vi "InitLinkButtons.vi"(5 "rightColumnAlignment":refnum<vi>, 6 "Col1Sec3_Top":refnum<vi>, 7 "leftColumnAlignment":refnum<vi>, 8 "icon array":refnum<vi>[](array[refnum]), 9 "button array":refnum<vi>[][](array[refnum]), 10 "item info array":T1(array[cluster]), 11 "Pnl Refnum":refnum<vi>) -> (3 "Handler info":variant)   [LabVIEW 2009, in "NavScreen.lvlib"]
uses:
  NavScreen.lvlib
  Classes/ClickableText/ClickableText.lvclass
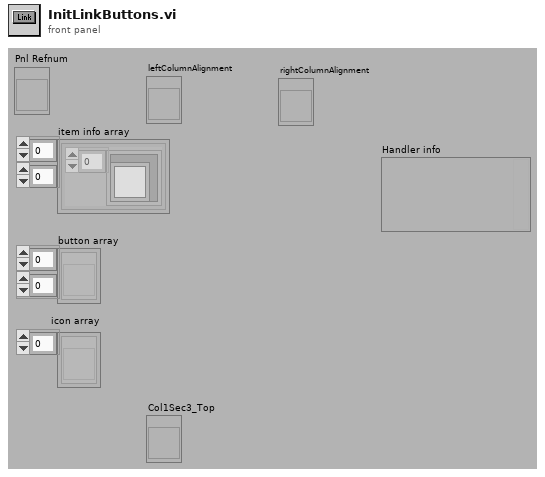
[diagram p1: front panel]
types:
  T1 = cluster{refnum<class "ClickableText.lvclass">[]}[][]
  T2 = typedef "NavScreen.lvlib/ItemData_Type.ctl" = enum16{"None", "Folder", "New Project", "New VI", "Find", "VI", "Project", "New from template", "RT Project Wizard", "PDA Project Wizard", "Control", "Library", "Class", "XControl", "Runtime menu"}
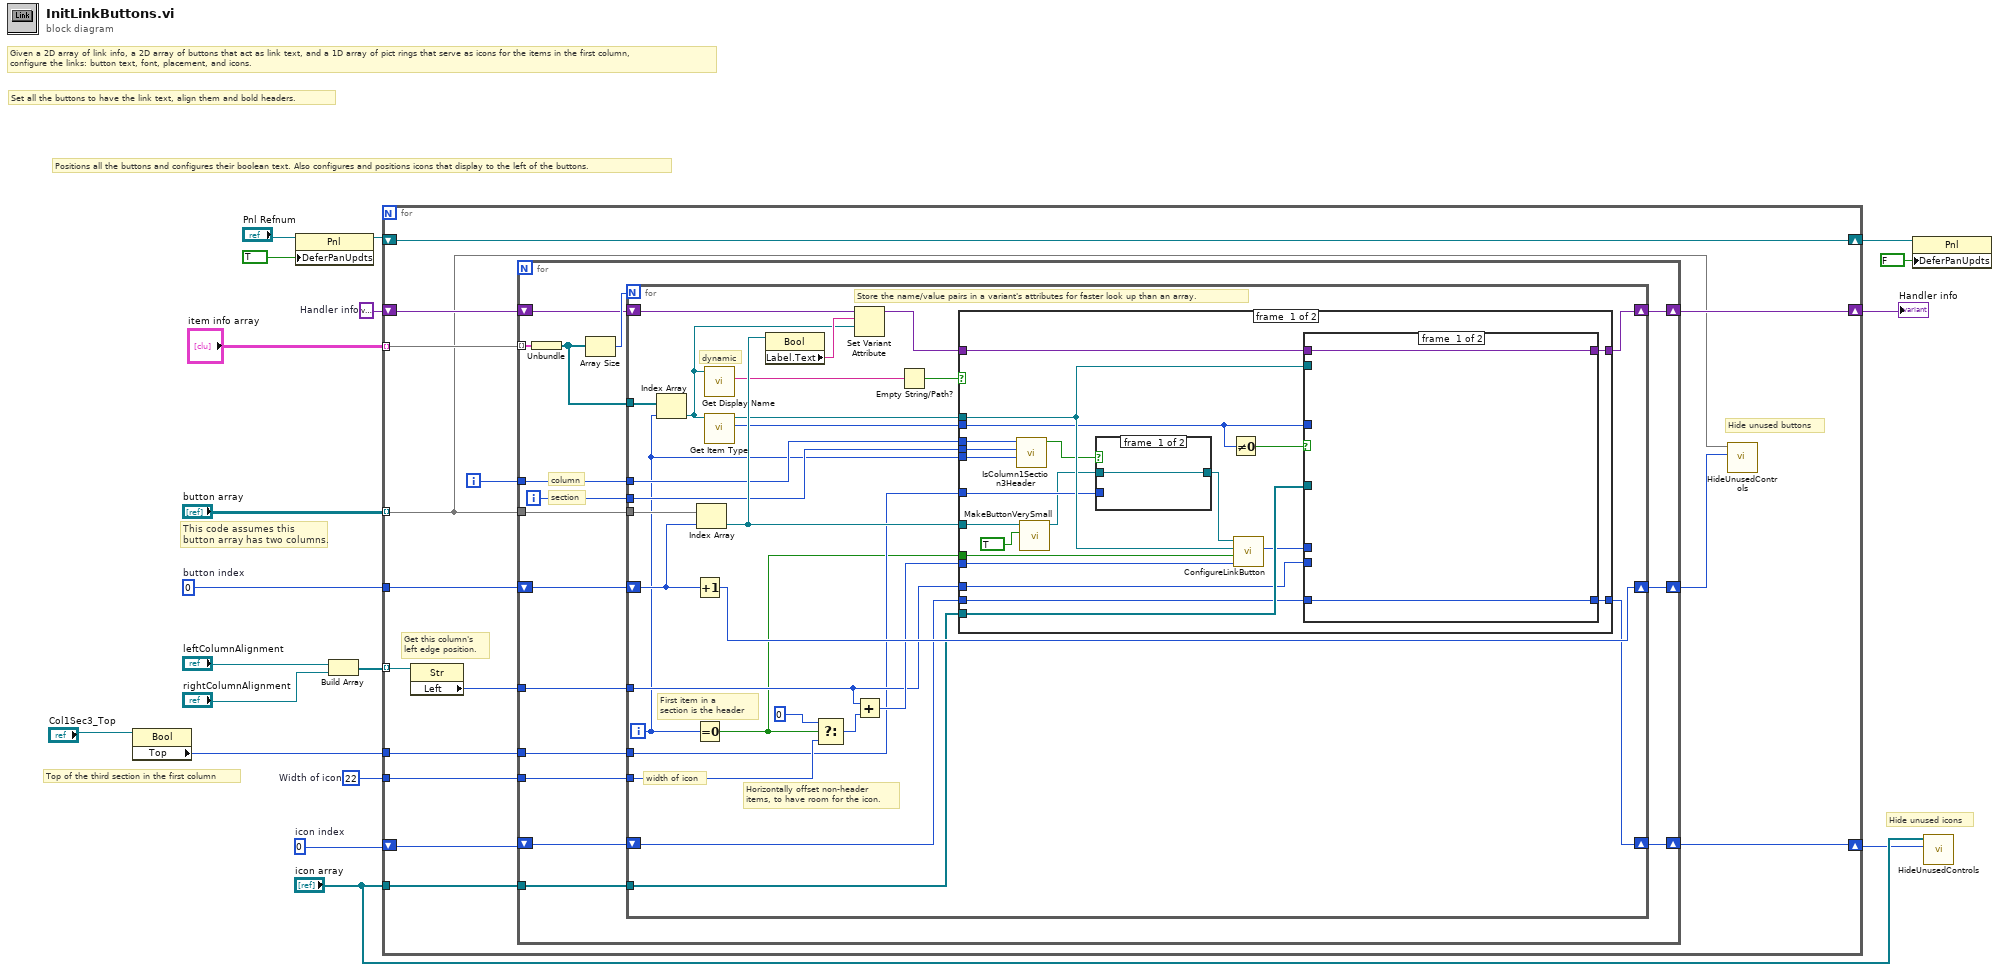
[diagram p0: block diagram]
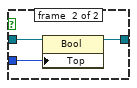
[diagram p2: hidden frame]
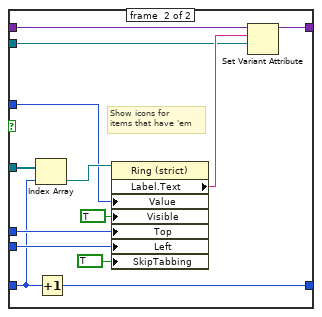
[diagram p3: hidden frame]
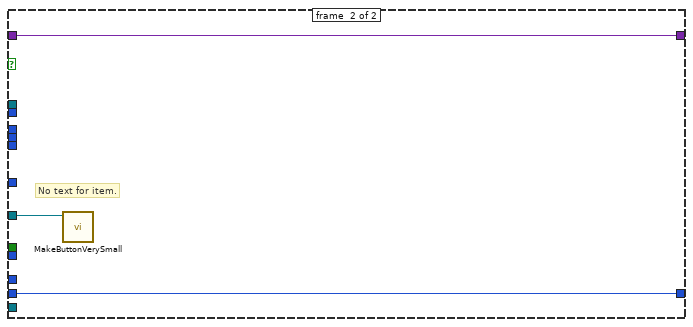
[diagram p4: hidden frame]
diagram:
  w2 = 0  # button index
  w4 = variant  # Handler info
  w9 = 22  # Width of icon
  w13 = 0  # icon index
  # "Positions all the buttons and configures their boolean text. Also configures and positions icons that display to the left of the buttons."
  # "Set all the buttons to have the link text, align them and bold headers."
  # "Top of the third section in the first column"
  # "Given a 2D array of link info, a 2D array of buttons that act as link text, and a 1D array of pict rings that serve as icons for the items in the first column,\nconfigure the links: button text, font, placement, and icons."
  # "This code assumes this\nbutton array has two columns."
  # "Hide unused icons"
  n1 = property on="Property Node" class="Bool"(reference="Col1Sec3_Top") -> ("Top"=w7:i32)  [unwired: 1 in, 2 out]
  n2 = property on="Property Node" class="Pnl"(reference="Pnl Refnum", "DeferPanUpdts"=TRUE ("Defer Panel Updates")) -> (reference out=w16:refnum<vi>)  [unwired: 1 in, 1 out]
  n3 = Build Array("leftColumnAlignment", "rightColumnAlignment") -> (w10:refnum<vi>[])
  n4 = for {
    tunnel: "button array" -> [w22] mode=indexing
    tunnel: "item info array" -> [w33] mode=indexing
    tunnel: "icon array" -> [w32]
    shift-right: [w30] -> w3
    shift-left: w4 -> [w31]
    shift-right: [w29] -> w14
    shift-left: w16 -> [w29]
    tunnel: w9 -> [w28]
    shift-right: [w26] -> w5
    shift-left: w13 -> [w27]
    tunnel: w10 -> [w25] mode=indexing
    tunnel: w7 -> [w24]
    tunnel: w2 -> [w20]
    i -> [w23]
    # "Get this column's\nleft edge position."
    # "Hide unused buttons"
    n5 = property on="Property Node" class="Str"(reference=w25) -> ("Left"=w34:i32)  [unwired: 1 in, 2 out]
    n6 = for {
      tunnel: w22 -> [w50]
      tunnel: w33 -> [w39] mode=indexing
      shift-right: [w48] -> w21
      shift-left: w20 -> [w49]
      tunnel: w34 -> [w47]
      shift-right: [w35] -> w30
      shift-left: w31 -> [w36]
      shift-right: [w45] -> w26
      shift-left: w27 -> [w46]
      tunnel: w32 -> [w44]
      tunnel: w28 -> [w43]
      tunnel: w24 -> [w42]
      tunnel: w23 -> [w41]
      i -> [w40]
      # "section"
      # "column"
      n7 = Unbundle(w39) -> (w37:refnum<class "ClickableText.lvclass">[])
      n8 = Array Size(array=w37) -> (size(s)=w38:i32)
      n9 = for {
        N: w38 -> [_]
        tunnel: w37 -> [w71]
        tunnel: w50 -> [w77]
        shift-right: [w75] -> w48
        shift-left: w49 -> [w76]
        tunnel: w47 -> [w66]
        shift-right: [w68] -> w45
        shift-left: w46 -> [w69]
        tunnel: w44 -> [w56]
        tunnel: w43 -> [w67]
        tunnel: w42 -> [w65]
        tunnel: w41 -> [w64]
        tunnel: w40 -> [w63]
        shift-right: [w51] -> w35
        shift-left: w36 -> [w57]
        i -> [w62]
        # "dynamic"
        # "First item in a\nsection is the header"
        # "Store the name/value pairs in a variant's attributes for faster look up than an array."
        # "width of icon"
        # "Horizontally offset non-header\nitems, to have room for the icon."
        n10 = Index Array(array=w71, index=w62) -> (element=w58:refnum<class "ClickableText.lvclass">)
        n11 = Increment(x=w76) -> (x+1=w75:i32)
        n12 = Equal To 0?(x=w62) -> (x = 0?=w54:bool)
        n13 = Index Array(array=w77, index=w76) -> (element=w70:refnum<vi>)
        n14 = call-dynamic "Get Display Name.vi"("ClickableText in"=w58) -> ("localized name"=w61:string)  [unwired: 8 in, 2 out]
        n15 = call "Get Item Type.vi"("ClickableText in"=w58) -> ("DNL_Type"=w60:T2, "ClickableText out"=w53:refnum<class "ClickableText.lvclass">)  [unwired: 8 in, 1 out]
        n16 = property on="Property Node" class="Bool"(reference=w70) -> ("Label.Text"=w59:string)  [unwired: 1 in, 2 out]
        n17 = Select(t=0, s=w54, f=w67) -> (s? t:f=w55:i32)
        n18 = Set Variant Attribute(Variant=w57, name=w59, value=w58) -> (Variant out=w52:variant)  [unwired: 1 in, 2 out]
        n19 = Add(x=w66, y=w55) -> (x+y=w74:i32)
        n20 = Empty String/Path?(string/path=w61) -> (empty?=w72:bool)
        n21 = case shown="False" w72 {
          tunnel: w74 -> [w80 _]
          tunnel: w70 -> [w90 w119]
          tunnel: w54 -> [w83 _]
          tunnel: w56 -> [w97 _]
          tunnel: w60 -> [w96 _]
          tunnel: w69 -> [w94 w120]
          tunnel: [w93 w120] -> w68
          tunnel: w66 -> [w81 _]
          tunnel: w65 -> [w92 _]
          tunnel: w64 -> [w87 _]
          tunnel: w63 -> [w86 _]
          tunnel: w62 -> [w85 _]
          tunnel: w53 -> [w98 _]
          tunnel: w52 -> [w79 w118]
          tunnel: [w78 w118] -> w51
          frame #0 {
            n22 = call "IsColumn1Section3Header.vi"("index 3"=w85, "index 2"=w86, "index 1"=w87) -> ("is col 1 section 3 header?"=w88:bool)  [unwired: 7 in, 1 out]
            n23 = call "MakeButtonVerySmall.vi"("visible"=TRUE ("Visible"), "Link Button 1"=w90) -> ("Link Button 2"=w89:refnum<vi>)  [unwired: 8 in, 1 out]
            n24 = case shown="True" w88 {
              tunnel: w89 -> [w99 w102]
              tunnel: [w99 w101] -> w84
              tunnel: w92 -> [_ w100]
              frame #0 {
              }
              frame #1 {
                n25 = property on="Property Node" class="Bool"(reference=w102, "Top"=w100) -> (reference out=w101:refnum<vi>)  [unwired: 1 in, 1 out]
              }
            }
            n26 = Not Equal To 0?(x=w96) -> (x != 0?=w95:bool)
            n27 = call "ConfigureLinkButton.vi"("Position:Left"=w80, "is section header?"=w83, "GettingStartedWindow.lvlib:ClickableText.lvclass"=w98, "Link Button 1"=w84) -> ("Top"=w82:i32)  [unwired: 6 in, 1 out]
            n28 = case shown="True" w95 {
              tunnel: w96 -> [_ w109]
              tunnel: w97 -> [_ w112]
              tunnel: w94 -> [w104 w110]
              tunnel: [w104 w116] -> w93
              tunnel: w82 -> [_ w115]
              tunnel: w81 -> [_ w114]
              tunnel: w79 -> [w103 w108]
              tunnel: w98 -> [_ w106]
              tunnel: [w103 w105] -> w78
              frame #0 {
              }
              frame #1 {
                # "Show icons for\nitems that have 'em"
                n29 = Index Array(array=w112, index=w110) -> (element=w111:refnum<vi>)
                n30 = Increment(x=w110) -> (x+1=w116:i32)
                n31 = property on="Property Node" class="Ring (strict)"(reference=w111, "Value"=w109, "Visible"=TRUE, "Top"=w115, "Left"=w114, "SkipTabbing"=TRUE ("Skip When Tabbing")) -> ("Label.Text"=w107:string)  [unwired: 1 in, 2 out]
                n32 = Set Variant Attribute(Variant=w108, name=w107, value=w106) -> (Variant out=w105:variant)  [unwired: 1 in, 2 out]
              }
            }
          }
          frame #1 {
            # "No text for item."
            n33 = call "MakeButtonVerySmall.vi"("Link Button 1"=w119) -> ()  [unwired: 9 in, 2 out]
          }
        }
      }
    }
    n34 = call "HideUnusedControls.vi"("last used index"=w21, "control array"=w22) -> ()  [unwired: 10 in]
  }
  "Handler info" <- w3
  n35 = property on="Property Node" class="Pnl"(reference=w14, "DeferPanUpdts"=FALSE ("Defer Panel Updates")) -> ()  [unwired: 1 in, 2 out]
  n36 = call "HideUnusedControls.vi"("last used index"=w5, "control array"="icon array") -> ()  [unwired: 10 in]
